vi "Read Combined Measured Value.vi"(8 "error in (no error)":errorcluster, 11 "VGC in":refnum<class "PL Inficon VGC.lvclass">) -> (0 "error out":errorcluster, 2 "measured value":dbl, 3 "VGC out":refnum<class "PL Inficon VGC.lvclass">)   [LabVIEW 2015, in "PL Inficon VGC.lvclass"]
doc: "Reads combined pressure range measured value."
uses:
  PL Inficon VGC.lvclass
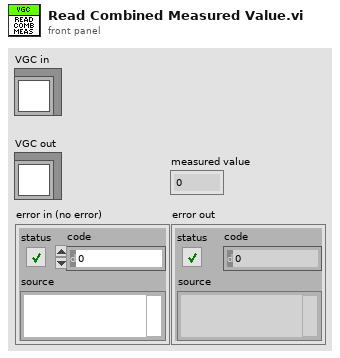
[diagram p1: front panel]
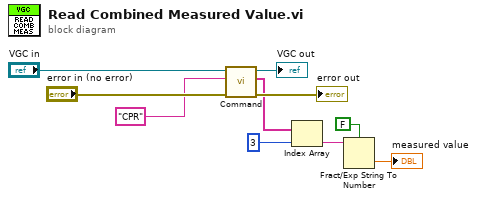
[diagram p0: block diagram]
diagram:
  n1 = call "Command.vi"("error in (no error)"="error in (no error)", "command"="CPR", "VGC in"="VGC in") -> ("error out"=→"error out":errorcluster, "response data"=w4:string[], "VGC out"=→"VGC out":refnum<class "PL Inficon VGC.lvclass">)  [unwired: 6 in]
  n2 = Index Array(array=w4, index=3) -> (element=w2:string)
  n3 = Fract/Exp String To Number(use system decimal point (T)=FALSE, string=w2) -> (number=→"measured value":dbl)  [unwired: 2 in, 1 out]
